vi "Set Spanfactors and Offests in Lin-Protocol.vi"(8 "error in (no error)":errorcluster caption="Fehler (Eingang, kein Fehler)", 11 "Lin-Polynom":T1 {"zusätzliche Zeitdauer Erster Punkt" format="%#_5g"; "Lin Modus" items=["Cal Gas to PNS", "Cal Gas to Samplepoint", "Measure"]; "Gas Ablaufdatum" format="%<%d.%m.%Y>T"; "HovaCAL Flow AutoLin"."HovaCAL Flow Input Cluster" format="%.2f"; "Gasflasche" items=["----"=10000, "IAG MG"=0, "IAG NH3 3000"=1, "IAG NH3 2000"=2, "IAG NH3 200"=3]; "Conditions:" items=["field", "laboratory"]; "Kalibrierauswahl" items=["Inaktiv", "Aktiv"]; "Anzahl Stufen" format="%#_5g"; "Zeitdauer Stufe" format="%#_5g"; "Verdünnungsgas" items=["N2", "O2"]; "Komponentenauswahl"."Konzentration" format="%#.6f"; "Gasnummer:" min=1 max=5; "Prüfgas Konzentration" format="%#.6f"; "Polynomkoeff." format="%#_18f"}) -> (0 "error out":errorcluster caption="Fehler (Ausgang)", 1 "Offset":sgl[](array[numeric]), 2 "Span":sgl[](array[numeric]), 3 "Lin-Polynom out":T1 {"zusätzliche Zeitdauer Erster Punkt" format="%#_5g"; "Lin Modus" items=["Cal Gas to PNS", "Cal Gas to Samplepoint", "Measure"]; "Gas Ablaufdatum" format="%<%d.%m.%Y>T"; "HovaCAL Flow AutoLin"."HovaCAL Flow Input Cluster" format="%.2f"; "Gasflasche" items=["----"=10000, "IAG MG"=0, "IAG NH3 3000"=1, "IAG NH3 2000"=2, "IAG NH3 200"=3]; "Conditions:" items=["field", "laboratory"]; "Kalibrierauswahl" items=["Inaktiv", "Aktiv"]; "Anzahl Stufen" format="%#_5g"; "Zeitdauer Stufe" format="%#_5g"; "Verdünnungsgas" items=["N2", "O2"]; "Komponentenauswahl"."Konzentration" format="%#.6f"; "Gasnummer:" min=1 max=5; "Prüfgas Konzentration" format="%#.6f"; "Polynomkoeff." format="%#_18f"})   [LabVIEW 2020, in "Linearisierung v2.lvlib"]
uses:
  Linearisierung v2.lvlib
  Lin-Polynom Daten.ctl
  KomponentenArray.ctl
  Visualisierungs Elemente/Auswahlfeld.ctl
  Visualisierungs Elemente/Zahlen-Eingabefeld.ctl
  EPA Optionsfeld.ctl
  Gasteiler/HovaCal/AutoLin Hovacal.ctl
  Kalibrieroption.ctl
  EPA1065-307/Condition.ctl
  Seiten/System Einstellungen V2/Konfig Gasflasche.ctl
  Seiten/System Einstellungen V2/Gasflasche Auswahl.ctl
  Gasteiler/HovaCAL_Interface/Controls/Flow Einstellung.ctl
  Gasteiler/HovaCAL_Interface/Controls/Pump state.ctl
  Seiten/CalGas Aufschaltung/Lin Modus.ctl
  Seiten/FT-IR/Span/Aktion FGV Span.ctl
  Seiten/FT-IR/Span/Spanfaktor.lvlib
  Gasteiler/Gasteiler.lvlib
  Gasteiler/HovaCal/HovaCal.lvlib
  EPA1065-307/Linearity verification 1065-307.lvlib
  Seiten/System Einstellungen V2/System Einstellungen V2.lvlib
  Gasteiler/HovaCAL_Interface/Controls/Controls.lvlib
  Seiten/CalGas Aufschaltung/CalGas Aufschaltung.lvlib
panel:
  # "%"
  # "%"
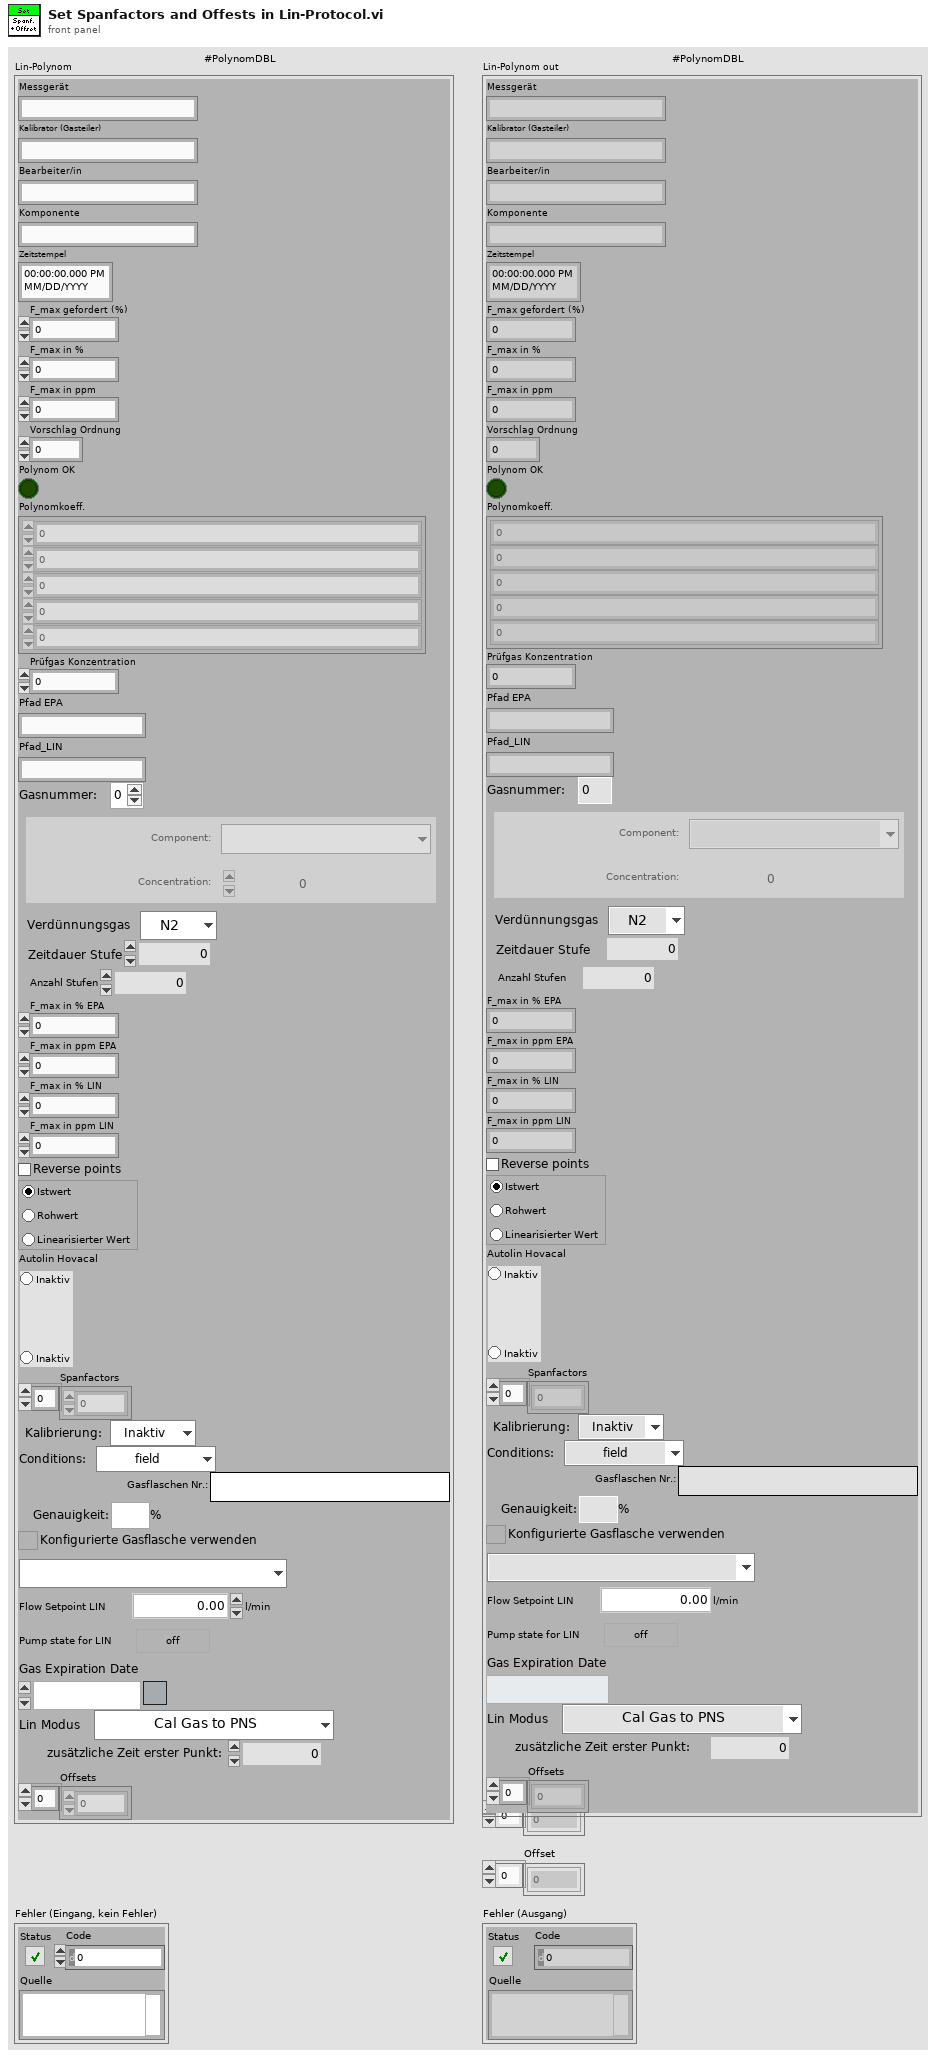
[diagram p1: front panel]
types:
  T1 = typedef "Linearisierung v2.lvlib/Lin-Polynom Daten.ctl" = cluster{"Messgerät":string, "Kalibrator (Gasteiler)":string, "Bearbeiter/in":string, "Komponente":string, "Zeitstempel":timestamp, "F_max gefordert (%)":sgl, "F_max in %":sgl, "F_max in ppm":sgl, "Vorschlag Ordnung":i32, "Polynom OK":bool, "Polynomkoeff.":dbl[], "Prüfgas Konzentration":dbl, "Pfad EPA":string, "Pfad_LIN":string, "Gasnummer:":u8, "Komponentenauswahl":T2, "Verdünnungsgas":T4, "Zeitdauer Stufe":T5, "Anzahl Stufen":T5, "F_max in % EPA":sgl, "F_max in ppm EPA":sgl, "F_max in % LIN":sgl, "F_max in ppm LIN":sgl, "Punkte umkehren":bool, "EPA Optionsfeld":T6, "Autolin Hovacal":T7, "Spanfactors":sgl[], "Kalibrierauswahl":T8, "Conditions:":T9, "Gasflaschen Nr.:":string, "Bottle Accuracy":dbl, "Konfig Gasflasche":T10, "Gasflasche":T11, "HovaCAL Flow AutoLin":T12, "MFC Output":T13, "Gas Ablaufdatum":timestamp, "Lin Modus":T14, "zusätzliche Zeitdauer Erster Punkt":sgl, "Offsets":sgl[]}
  T2 = typedef "Linearisierung v2.lvlib/KomponentenArray.ctl" = cluster{"Komponente:":T3, "Konzentration":dbl}[]
  T3 = typedef "Auswahlfeld.ctl" = u16
  T4 = typedef "Linearisierung v2.lvlib/Gasteiler.lvlib/Prüfgas in.ctl" = u16
  T5 = typedef "Zahlen-Eingabefeld.ctl" = sgl
  T6 = typedef "Linearisierung v2.lvlib/EPA Optionsfeld.ctl" = enum32{"Istwert", "Rohwert", "Linearisierter Wert"}
  T7 = typedef "Linearisierung v2.lvlib/Gasteiler.lvlib/HovaCal.lvlib/AutoLin Hovacal.ctl" = enum32{"Keine Auswahl", "Optionsauswahl 1", "Optionsauswahl 2"}
  T8 = typedef "Linearisierung v2.lvlib/Kalibrieroption.ctl" = u16
  T9 = typedef "Linearisierung v2.lvlib/Linearity verification 1065-307.lvlib/Condition.ctl" = u16
  T10 = typedef "System Einstellungen V2.lvlib/Konfig Gasflasche.ctl" = bool
  T11 = typedef "System Einstellungen V2.lvlib/Gasflasche Auswahl.ctl" = u16
  T12 = typedef "Linearisierung v2.lvlib/Gasteiler.lvlib/HovaCAL_Interface.lvlib/Controls.lvlib/Flow Einstellung.ctl" = cluster{"HovaCAL Flow Input Cluster":dbl}
  T13 = typedef "Linearisierung v2.lvlib/Gasteiler.lvlib/HovaCAL_Interface.lvlib/Controls.lvlib/Pump state.ctl" = cluster{"Run":bool}
  T14 = typedef "CalGas Aufschaltung.lvlib/Lin Modus.ctl" = u16
  T15 = typedef "FT-IR.lvlib/Spanfaktor.lvlib/Aktion FGV Span.ctl" = enum16{"lesen", "Span", "Seite aktiv", "Offset", "FGV aktualisiert", "Aktualisierung aufheben"}
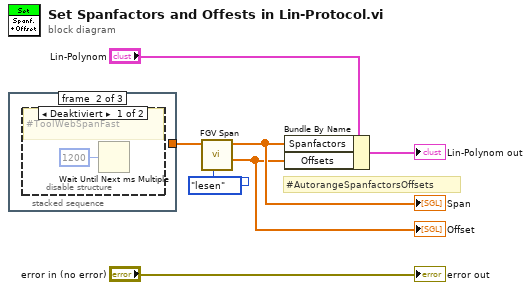
[diagram p0: block diagram]
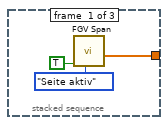
[diagram p2: hidden frame]
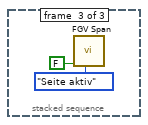
[diagram p4: hidden frame]
diagram:
  # "#AutorangeSpanfactorsOffsets"
  n1 = stacked-sequence {
    tunnel: [w8 _ _] -> w3
    frame #0 {
      n2 = call "FGV Span.vi"("Aktion"=Aktion_FGV_Span."Seite aktiv", "Aktiv"=TRUE) -> ("Offset"=w8:sgl[])  [unwired: 6 in, 3 out]
    }
    frame #1 {
      n3 = disable-structure shown="Deaktiviert" {
        frame Disabled {
          # "#ToolWebSpanFast"
          n4 = Wait Until Next ms Multiple(millisecond multiple=u32 1200 ("ms")) -> ()  [unwired: 1 out]
        }
        frame Enabled {
        }
      }
    }
    frame #2 {
      n5 = call "FGV Span.vi"("Aktion"=Aktion_FGV_Span."Seite aktiv", "Aktiv"=FALSE) -> ()  [unwired: 6 in, 4 out]
    }
  }
  n6 = call "FGV Span.vi"("Aktion"=Aktion_FGV_Span."lesen", "Span"=w3) -> ("Offset"=w1:sgl[], "Span"=w7:sgl[])  [unwired: 6 in, 2 out]
  "Offset" <- w1
  "Span" <- w7
  n7 = Bundle By Name(cluster="Lin-Polynom", "Spanfactors"=w7, "Offsets"=w1) -> (→"Lin-Polynom out":T1)
  "error out" <- "error in (no error)"
